vi "Generate Hologram.vi"(0 "x":sgl[](array[numeric]), 1 "y":sgl[](array[numeric]), 2 "z":sgl[](array[numeric]), 3 "spot_intensities":sgl[](array[numeric]), 4 "CUDA/SLM error in":errorcluster, 5 "alpha RPC":sgl=1.0, 9 "N_iterations":i32, 10 "method":i32, 12 "CGH in":u8[][](array[numeric])=array512x512[262144 elements]) -> (24 "CGH out":u8[][](array[numeric]), 25 "weights":sgl[][](graph)=[[0.32087266, 0.30867794, 0.31952837, 0.32111803, 0.32117248, 0.3210771, 0.32099402, 0.32094038, 0.32090643, 0.32088554], [0.32087216, 0.30864686, 0.31954217, 0.32109785, 0.3211845, 0.32108435, 0.32099703, 0.32094118, 0.3209064, 0.32088524], [0.32087475, 0.30863738, 0.3195775, 0.3210921, 0.32118624, 0.3210818, 0.32099742, 0.32094282, 0.32090908, 0.32088798], [0.3208743, 0.3086348, 0.31957102, 0.3210825, 0.3211723, 0.32108226, 0.32100248, 0.3209465, 0.3209109, 0.3208884], [0.32082918, 0.33360976, 0.32222247, 0.3205971, 0.32050273, 0.32060897, 0.32069725, 0.32075626, 0.3207928, 0.3208153], [0.3208285, 0.33361444, 0.32216293, 0.32054555, 0.32047704, 0.3205865, 0.32068458, 0.32074872, 0.32078892, 0.32081345], [0.3208247, 0.333552, 0.32235736, 0.32059258, 0.32051176, 0.32061282, 0.32069716, 0.32075158, 0.32078704, 0.3208098], [0.3208295, 0.33357766, 0.32223862, 0.32057458, 0.32048234, 0.32059732, 0.32069272, 0.3207548, 0.32079253, 0.3208156]], 27 "CUDA/SLM error out":errorcluster)   [LabVIEW 8.6]
uses:
  GenerateHologramCUDA.dll
panel:
  out "weights":sgl[](array[numeric])
  out "return":sgl
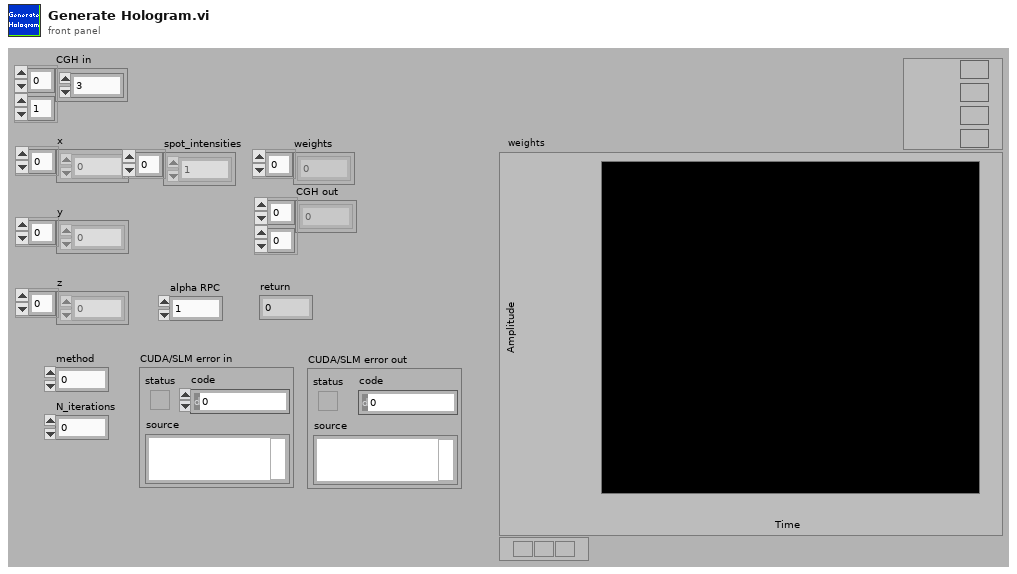
[diagram p1: front panel]
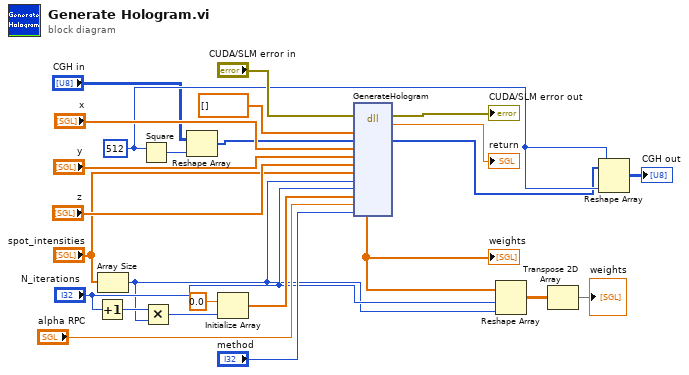
[diagram p0: block diagram]
diagram:
  w6 = 512 ("SLM size")
  n1 = Increment(x="N_iterations") -> (x+1=w17:i32)
  n2 = Array Size(array="spot_intensities") -> (size(s)=w8:i32)
  n3 = Square(x=w6) -> (x^2=w7:i32)
  n4 = Multiply(x=w17, y=w8) -> (x*y=w16:i32)
  n5 = Reshape Array("CGH in", w7) -> (w5:u8[])
  n6 = Initialize Array(sgl 0.0 ("element"), w16) -> (w14:sgl[])
  n7 = dll-call lib="C:/Users/Martin/Dropbox/GU/CUDA/GenerateHologramCUDA/LabVIEW/GenerateHologramCUDA.dll" fn="GenerateHologram"(error in="CUDA/SLM error in", "V"=sgl[] [], "h_pSLM"=w5, "x"="x", "y"="y", "z"="z", "spot_amplitudes"="spot_intensities", "N_spots"=w8, "N_iterations"="N_iterations", "weights"=w14, "alpha"="alpha RPC", "method"="method") -> (error out=→"CUDA/SLM error out":errorcluster, "return"=→"return":sgl, "h_pSLM"=w2:u8[], "weights"=w10:sgl[])  [unwired: 6 in, 6 out]
  "weights" <- w10
  n8 = Reshape Array(w10, "N_iterations", w8) -> (w12:sgl[][])
  n9 = Transpose 2D Array(2D array=w12) -> (transposed array=→"weights":sgl[][])
  n10 = Reshape Array(w2, w6, w6) -> (→"CGH out":u8[][])
